vi "Match 1D Array Elements - boolean.vi"(1 "mode (any)":enum16{"any", "each"}(ring)=enum."each", 2 "elements (none)":bool[](array[boolean]), 3 "1D Array":bool[](array[boolean])) -> (0 "indices":i32[](array[numeric]))   [LabVIEW 2020]
doc: "Searches through a 1D array for the list of elements. In the \"any\" mode, the 1D array is searched once for elements matching any contained in the list of elements. In the \"each\" mode this is a list-based version of the built-in \"Search 1D Array\". Neither the 1D array or the list of elements to be found need be sorted."
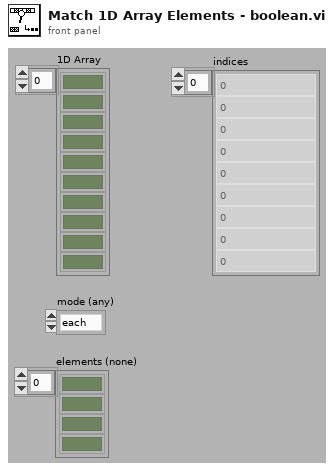
[diagram p1: front panel]
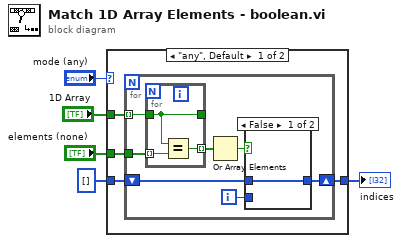
[diagram p0: block diagram]
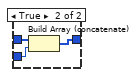
[diagram p2: hidden frame]
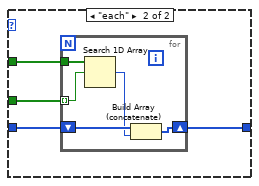
[diagram p3: hidden frame]
diagram:
  n1 = case shown="\"any\", Default" "mode (any)" {
    tunnel: "1D Array" -> [w9 w27]
    tunnel: "elements (none)" -> [w8 w26]
    tunnel: [w7 w25] -> w3
    tunnel: i32[] [] ("indices (none)") -> [w6 w24]
    frame "any", Default {
      n2 = for {
        tunnel: w9 -> [w15] mode=indexing
        tunnel: w8 -> [w16]
        shift-right: [w13] -> w7
        shift-left: w6 -> [w12]
        i -> [w11]
        n3 = for {
          tunnel: w16 -> [w19] mode=indexing
          tunnel: w15 -> [w17]
          tunnel: [w18] -> w10 mode=indexing
          tunnel: [w17] -> _
          n4 = Equal?(x=w17, y=w19) -> (x = y?=w18:bool)
        }
        n5 = Or Array Elements(Boolean array=w10) -> (logical OR=w14:bool)
        n6 = case shown="False" w14 {
          tunnel: [w20 w23] -> w13
          tunnel: w12 -> [w20 w22]
          tunnel: w11 -> [_ w21]
          frame False {
          }
          frame True {
            n7 = Build Array (concatenate)(w22, w21) -> (w23:i32[])
          }
        }
      }
    }
    frame "each" {
      n8 = for {
        tunnel: w27 -> [w32]
        tunnel: w26 -> [w31] mode=indexing
        shift-right: [w29] -> w25
        shift-left: w24 -> [w30]
        n9 = Search 1D Array(1D array=w32, element=w31) -> (index of element=w28:i32)  [unwired: 1 in]
        n10 = Build Array (concatenate)(w30, w28) -> (w29:i32[])
      }
    }
  }
  "indices" <- w3
